vi "未命名 1.vi"() -> ()   [LabVIEW 2018]
uses:
  <vilib>/Utility/NIReport.llb/Report Type.ctl
  <vilib>/Utility/NIReport.llb/NI_ReportGenerationCore.lvlib
panel:
  out "检查文件路径是否正确 2":bool caption="文件或文件夹存在？"
  out "保存路径 2":path
  in  "产品序号 2":string
  in  "部位 2":string="位置1"
  in  "类型 2":string="类型1"
  in  "合格性 2":string="合格"
  in  "检验人 2":string
  out "模板路径 2":path
  in  "报告生成":bool
  out "Particle Measurements (Pixels) 2":dbl[][](array[numeric]) format="%.2f"
  out "检查文件路径是否正确":bool caption="文件或文件夹存在？"
  out "保存路径":path
  in  "产品序号":string
  in  "部位":string="位置1"
  in  "类型":string="类型1"
  in  "合格性":string="合格"
  in  "检验人":string
  out "模板路径":path
  out "Particle Measurements (Pixels)":dbl[][](array[numeric]) format="%.2f"
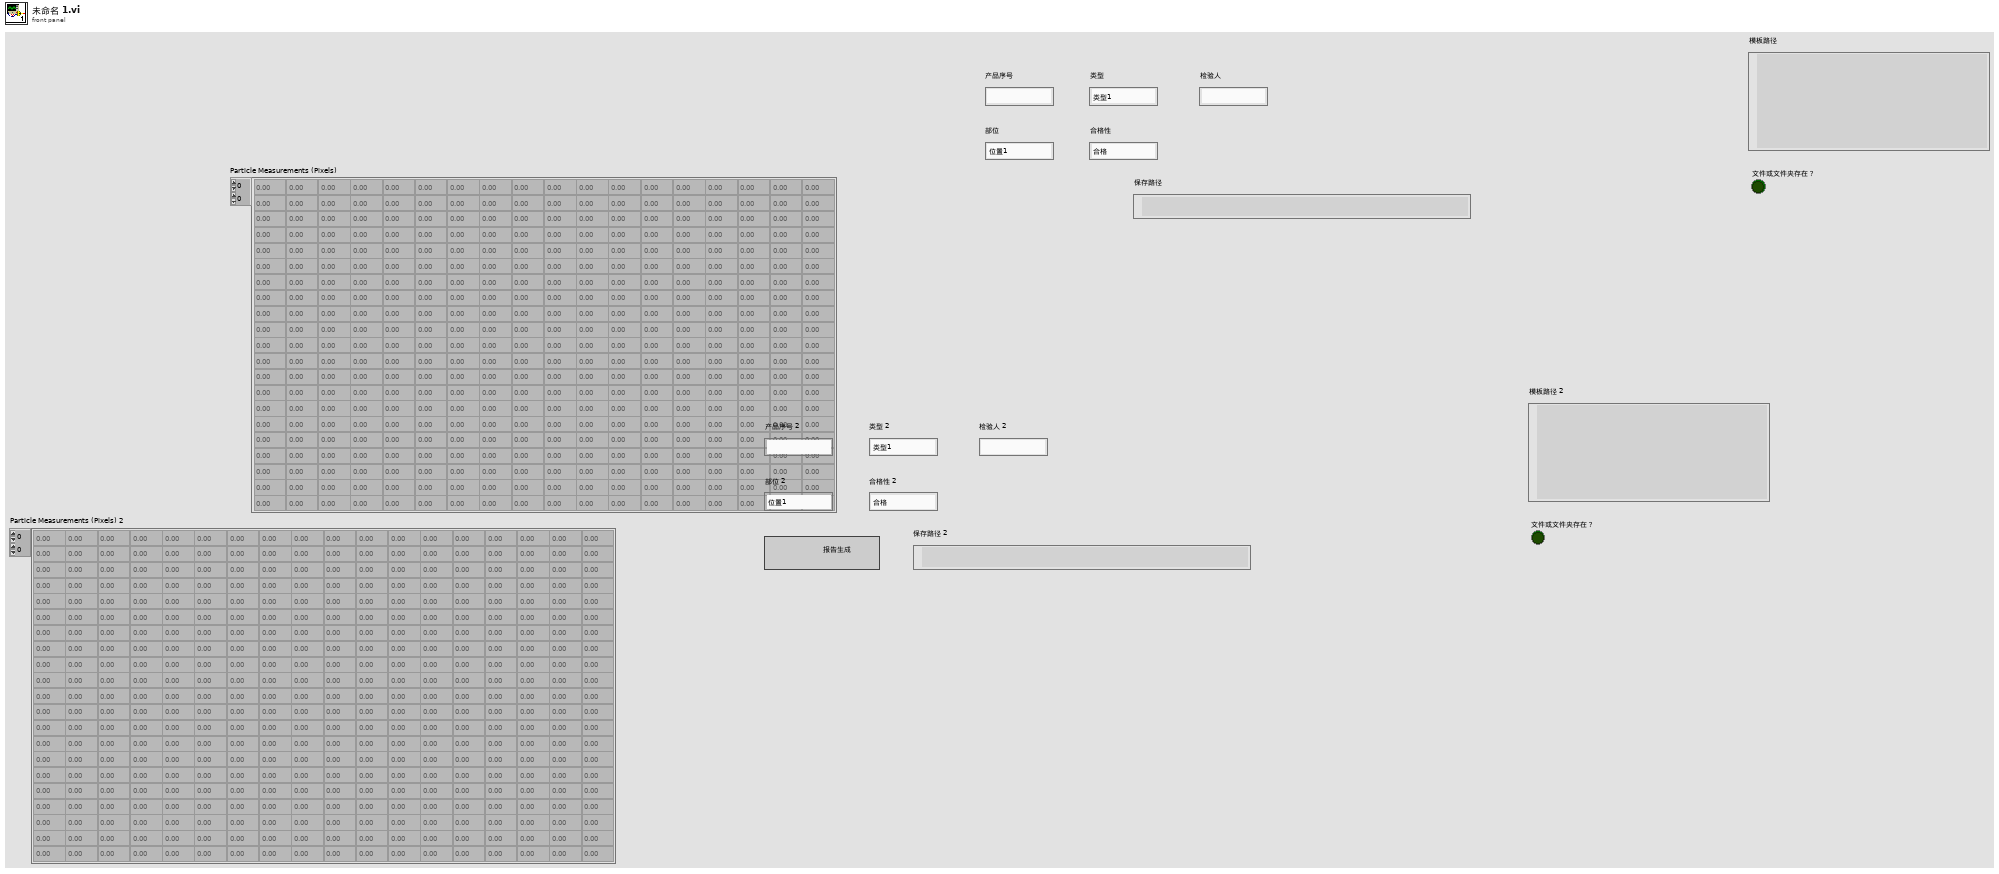
[diagram p1: front panel]
types:
  T1 = typedef "NI_ReportGenerationCore.lvlib/Report Type.ctl" = enum16{"HTML", "Word", "Excel"}
  T2 = cluster{"position (excel)":cluster{"row":i32, "column":i32}, "name (excel)":string, "bookmark (word)":string}
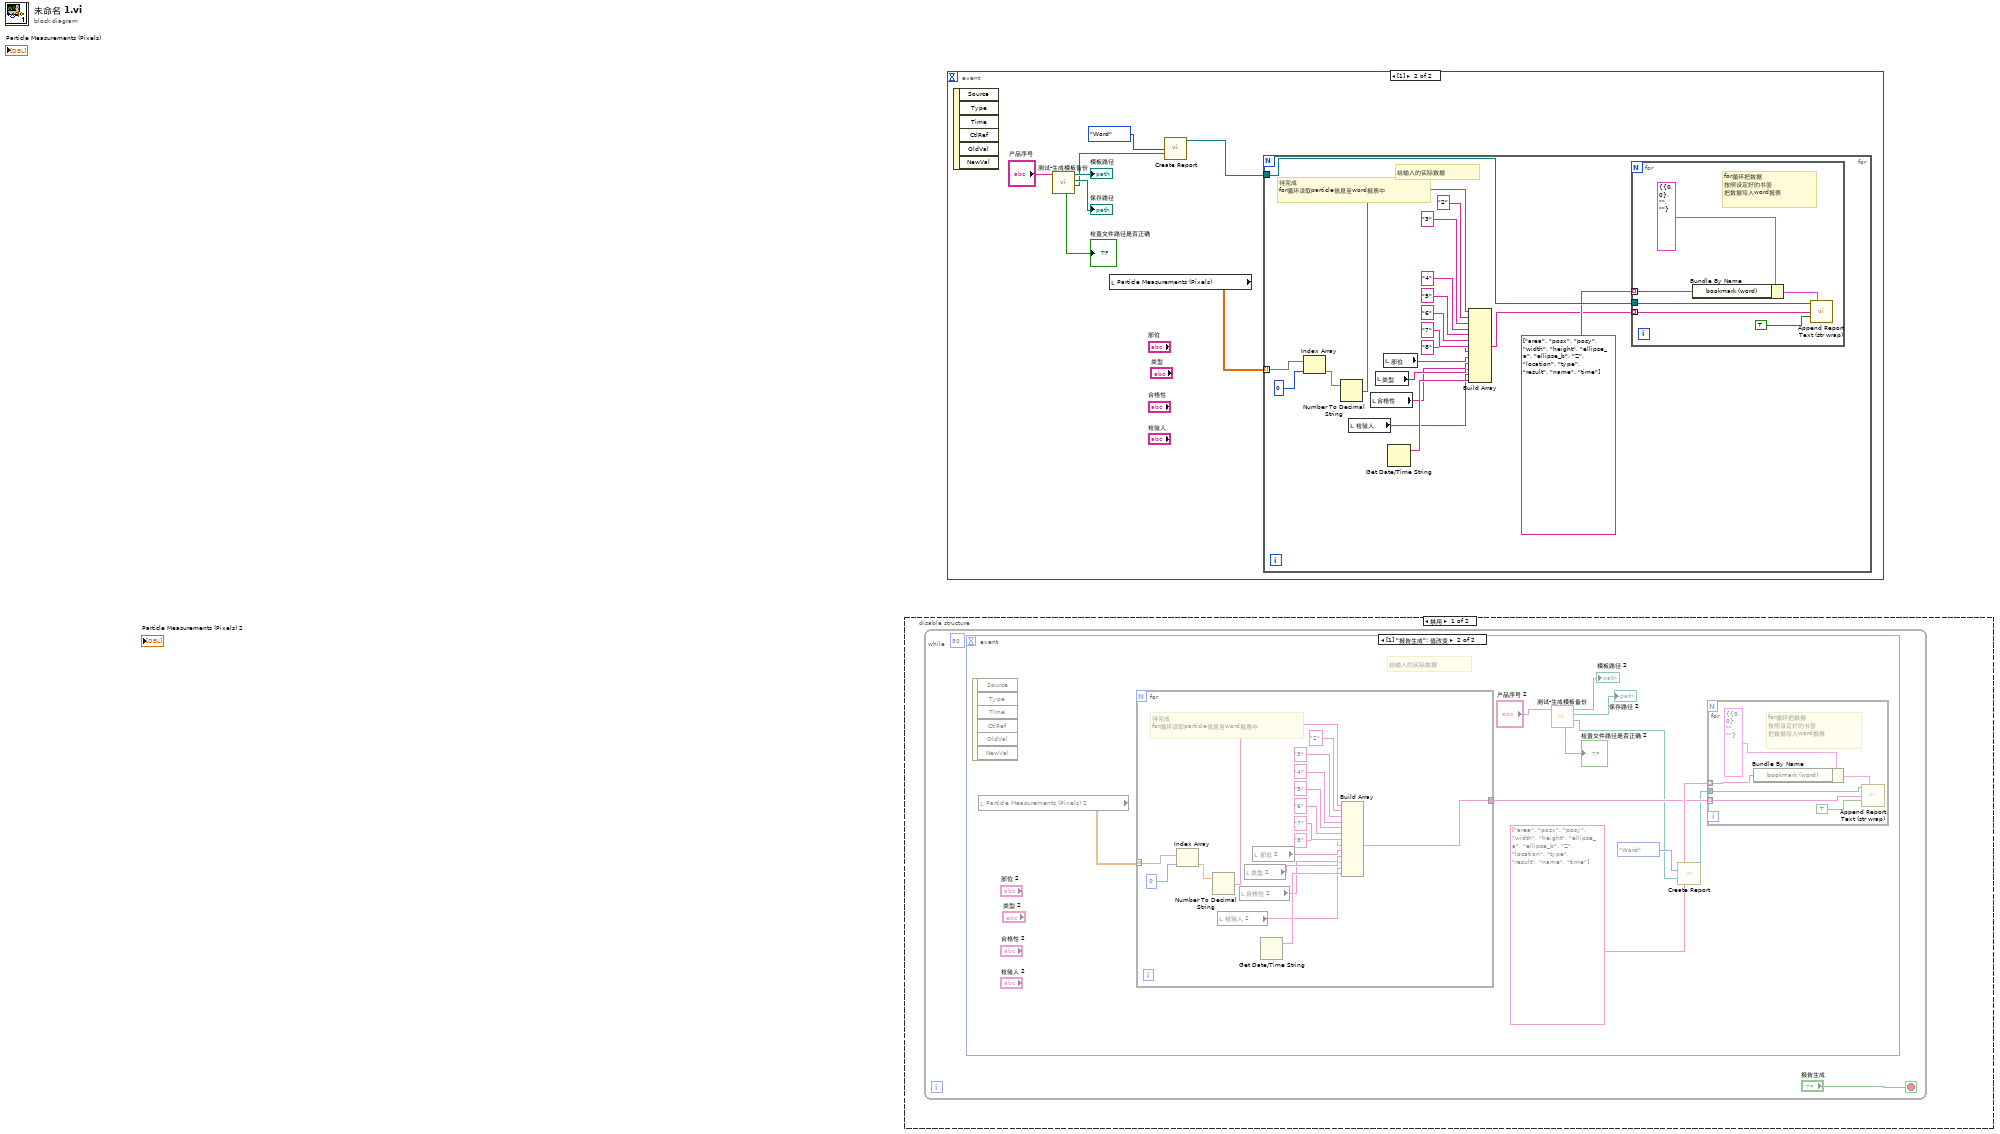
[diagram p0: block diagram]
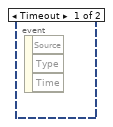
[diagram p2: hidden frame]
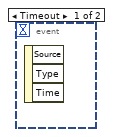
[diagram p4: hidden frame]
diagram:
  n1 = disable-structure shown="禁用" {
    frame Disabled {
      n2 = while {
        stop <- "报告生成" stop-if-true
        (unwired) 50
        n3 = event shown="[1] \"报告生成\": 值改变" {
          selector: _ -> [_ _]
          dyn-events: _ -> [_ _]
          timeout: _ -> [_ _]
          event Timeout {
            n4 = event-data() -> ()  [unwired: 1 in, 3 out]
          }
          event "报告生成": Value Change {
            # "给输入的实际数据"
            n5 = event-data() -> ()  [unwired: 1 in, 6 out]
            n6 = local read "Particle Measurements (Pixels) 2"() -> (w2:dbl[][])
            n7 = for {
              tunnel: [w25] -> w10
              tunnel: w2 -> [w19] mode=indexing
              # "待完成\nfor循环读取particle信息至word报表中"
              n8 = Index Array(array=w19, index=0 ("索引 (行)")) -> (element=w12:dbl)
              n9 = Number To Decimal String(number=w12) -> (decimal integer string=w17:string)  [unwired: 1 in]
              n10 = local read "检验人 2"() -> (w13:string)
              n11 = local read "合格性 2"() -> (w14:string)
              n12 = local read "类型 2"() -> (w15:string)
              n13 = local read "部位 2"() -> (w16:string)
              n14 = Get Date/Time String() -> (date string=w20:string)  [unwired: 3 in, 1 out]
              n15 = Build Array(w17, "2", "3", "4", "5" ("元素"), "6" ("元素"), "7" ("元素"), "8" ("元素"), w16, w15, w14, w13, w20) -> (w25:string[])
            }
            n16 = call "测试-生成模板备份.vi"("输入产品序号"="产品序号 2") -> ("new path"=w4:path, "保存路径"=→"保存路径 2":path, "模板路径"=→"模板路径 2":path, "检查文件路径是否正确"=→"检查文件路径是否正确 2":bool)  [unwired: 7 in]
            n17 = call "Create Report.vi"("report type"=Report_Type."Word", "template (empty)"=w4) -> ("report out"=w3:refnum<class "NI_report.lvclass">)  [unwired: 12 in, 1 out]
            n18 = for {
              tunnel: w3 -> [w32]
              tunnel: string[] ["area", "posx", "posy", "width", "height", "ellipse_a", "ellipse_b", "Z", "location", "type", "result", "name", "time"] -> [w33] mode=indexing
              tunnel: w10 -> [w31] mode=indexing
              # "for循环把数据\n按照设定好的书签 \n把数据写入word报表"
              n19 = Bundle By Name(cluster=T2 {"position (excel)"={"row"=0, "column"=0}, "name (excel)"="", "bookmark (word)"=""} ("MS Office parameters"), "bookmark (word)"=w33) -> (w30:T2)
              n20 = call "Append Report Text (str wrap).vi"("report in"=w32, "MS Office parameters"=w30, "text"=w31, "append on new line? (F)"=TRUE) -> ()  [unwired: 8 in, 4 out]
            }
          }
        }
      }
    }
    frame Enabled {
    }
  }
  n21 = event shown="[1]" {
    selector: _ -> [_ _]
    dyn-events: _ -> [_ _]
    timeout: _ -> [_ _]
    event Timeout {
      n22 = event-data() -> ()  [unwired: 1 in, 3 out]
    }
    event #1 (no event record) {
      n23 = event-data() -> ()  [unwired: 1 in, 6 out]
      n24 = call "测试-生成模板备份.vi"("输入产品序号"="产品序号") -> ("new path"=w37:path, "保存路径"=→"保存路径":path, "模板路径"=→"模板路径":path, "检查文件路径是否正确"=→"检查文件路径是否正确":bool)  [unwired: 7 in]
      n25 = local read "Particle Measurements (Pixels)"() -> (w36:dbl[][])
      n26 = call "Create Report.vi"("report type"=Report_Type."Word", "template (empty)"=w37) -> ("report out"=w35:refnum<class "NI_report.lvclass">)  [unwired: 12 in, 1 out]
      n27 = for {
        tunnel: w36 -> [w53] mode=indexing
        tunnel: w35 -> [w45]
        # "给输入的实际数据"
        # "待完成\nfor循环读取particle信息至word报表中"
        n28 = Index Array(array=w53, index=0 ("索引 (行)")) -> (element=w46:dbl)
        n29 = Number To Decimal String(number=w46) -> (decimal integer string=w51:string)  [unwired: 1 in]
        n30 = local read "检验人"() -> (w47:string)
        n31 = local read "合格性"() -> (w48:string)
        n32 = local read "类型"() -> (w49:string)
        n33 = local read "部位"() -> (w50:string)
        n34 = Get Date/Time String() -> (date string=w54:string)  [unwired: 3 in, 1 out]
        n35 = Build Array(w51, "2", "3", "4", "5" ("元素"), "6" ("元素"), "7" ("元素"), "8" ("元素"), w50, w49, w48, w47, w54) -> (w43:string[])
        n36 = for {
          tunnel: w45 -> [w64]
          tunnel: string[] ["area", "posx", "posy", "width", "height", "ellipse_a", "ellipse_b", "Z", "location", "type", "result", "name", "time"] -> [w63] mode=indexing
          tunnel: w43 -> [w62] mode=indexing
          # "for循环把数据\n按照设定好的书签 \n把数据写入word报表"
          n37 = Bundle By Name(cluster=T2 {"position (excel)"={"row"=0, "column"=0}, "name (excel)"="", "bookmark (word)"=""} ("MS Office parameters"), "bookmark (word)"=w63) -> (w67:T2)
          n38 = call "Append Report Text (str wrap).vi"("report in"=w64, "MS Office parameters"=w67, "text"=w62, "append on new line? (F)"=TRUE) -> ()  [unwired: 8 in, 4 out]
        }
      }
    }
  }
